vi "S4GUI_002.vi"(7 "Tab ObsEng":enum32{"Obs", "CCD modes", "Eng"}(tab)) -> ()   [LabVIEW 2018] (continued)
    tunnel: [_ _ _ w73] -> w5
    frame #0 {
      w37 = T12."Disabled and Grayed Out" ("Disabled")
      (unwired) u32 240 ("Tab Control Pane Dimension:Width")
      (unwired) u32 300 ("Tab Control Pane Dimension:Height")
      n2 = disable-structure shown="Enabled" {
        disable-tunnel: u32 211 ("Tab Control Pane Dimension:Height") -> [w46 _]
        disable-tunnel: u32 225 ("Tab Control Pane Dimension:Width") -> [w45 _]
        disable-tunnel: w36 -> [w44 _]
        disable-tunnel: w36 -> [w43 _]
        disable-tunnel: w36 -> [w42 _]
        disable-tunnel: w36 -> [w41 _]
        frame Enabled {
          n3 = property on="Tab CH1" class="TabCtl (strict)"(error in=w44, "PaneHeight"=w46, "PaneWidth"=w45) -> ()  [unwired: 1 in, 2 out]
          n4 = property on="Tab CH2" class="TabCtl (strict)"(error in=w43, "PaneHeight"=w46, "PaneWidth"=w45) -> ()  [unwired: 1 in, 2 out]
          n5 = property on="Tab CH3" class="TabCtl (strict)"(error in=w42, "PaneHeight"=w46, "PaneWidth"=w45) -> ()  [unwired: 1 in, 2 out]
          n6 = property on="Tab CH4" class="TabCtl (strict)"(error in=w41, "PaneHeight"=w46, "PaneWidth"=w45) -> ()  [unwired: 1 in, 2 out]
        }
        frame Disabled {
        }
      }
      n7 = local write "loop max(ms)"(u32 0 ("loop max(ms)")) -> ()
      n8 = property on="Set from Input ch1" class="Bool"(error in=w36, "DisabledEnum"=w37) -> ()  [unwired: 1 in, 2 out]
      n9 = property on="Set from Input ch3" class="Bool"(error in=w36, "DisabledEnum"=w37) -> ()  [unwired: 1 in, 2 out]
      n10 = property on="Set from Input ch2" class="Bool"(error in=w36, "DisabledEnum"=w37) -> ()  [unwired: 1 in, 2 out]
      n11 = property on="Set from Input ch4" class="Bool"(error in=w36, "DisabledEnum"=w37) -> (error out=w35:errorcluster)  [unwired: 1 in, 1 out]
    }
    frame #1 {
      w48 = u16 0 items=["OFF", "Lambda/2", "Lambda/4"] ("Lambda Selector")
      w52 = TRUE ("CH1on")
      w56 = u16 1 items=["Asynchronous", "Synchronous by Cycle"] ("SSM")
      w55 = u16 4 items=["All 16 positions", "First 8 positions", "First 4 positions", "1-4 & 9-12", "Clear", "Customized"] ("Select Positions")
      n12 = property on="#Pol. Seq. Done" class="Slide (strict)"(error in=w51, "Scale.Maximum"=0.0 ("Scale.Range:Maximum"), "Scale.Minimum"=0.0 ("Scale.Range:Minimum")) -> (error out=w50:errorcluster)  [unwired: 1 in, 1 out]
      n13 = local write "Tab ObsEng"(enum32{"Obs", "CCD modes", "Eng"}."Obs" ("Tab ObsEng")) -> ()
      n14 = property on="Tab ObsEng" class="TabCtl (strict)"(error in=w51, "Visible"=TRUE) -> ()  [unwired: 1 in, 2 out]
      n15 = property on="S4ICS protocol" class="Bool (strict)"(error in=w51, "Value"=FALSE ("S4ICS protocol"), "DisabledEnum"=T12."Disabled and Grayed Out" ("Disabled")) -> ()  [unwired: 1 in, 2 out]
      n16 = property on="SSM" class="Ring (strict)"(error in=w51, "Value"=w56) -> ()  [unwired: 1 in, 2 out]
      n17 = property on="TCS mode" class="Bool (strict)"(error in=w51, "Value"=TRUE ("TCS mode"), "DisabledEnum"=T12."Disabled and Grayed Out" ("Disabled")) -> ()  [unwired: 1 in, 2 out]
      n18 = property on="Lambda Selector" class="Ring (strict)"("Value"=w48) -> (error out=w49:errorcluster)  [unwired: 2 in, 1 out]
      n19 = local write "Select Positions"(w55) -> ()
      n20 = local write "password 2"("" ("password")) -> ()
      n21 = local write "password"("" ("password")) -> ()
      n22 = local write "CH2on"(w52) -> ()
      n23 = local write "CH3 on"(w52) -> ()
      n24 = local write "CH4 on"(w52) -> ()
      n25 = local write "CH1on"(w52) -> ()
      n26 = property on="Lambda Selector" class="Ring (strict)"(error in=w49, "RingText.Text"="Select...") -> ()  [unwired: 1 in, 2 out]
    }
    frame #2 {
      w69 = FALSE
      w66 = FALSE ("Cooler status 1")
      w65 = "" ("Temp Status 1")
      w70 = i16 0 ("Curr Temp 1")
      n27 = local write "Cooler status 4"(w66) -> ()
      n28 = local write "Curr Temp 4"(w70) -> ()
      n29 = local write "Panel Temp 4"(w70) -> ()
      n30 = local write "Temp Status 4"(w65) -> ()
      n31 = local write "Panel cooler 1"(w66) -> ()
      n32 = local write "Panel cooler 4"(w66) -> ()
      n33 = local write "Cooler status 1"(w66) -> ()
      n34 = local write "Curr Temp 1"(w70) -> ()
      n35 = local write "Panel Temp"(w70) -> ()
      n36 = local write "Temp Status 1"(w65) -> ()
      n37 = local write "Temp Status 3"(w65) -> ()
      n38 = local write "Panel Temp 3"(w70) -> ()
      n39 = local write "Panel cooler 2"(w66) -> ()
      n40 = local write "Curr Temp 2"(w70) -> ()
      n41 = local write "Panel Temp 2"(w70) -> ()
      n42 = local write "Temp Status 2"(w65) -> ()
      n43 = local write "Panel cooler 3"(w66) -> ()
      n44 = local write "Cooler status 3"(w66) -> ()
      n45 = local write "Cooler status 2"(w66) -> ()
      n46 = local write "Curr Temp 3"(w70) -> ()
      n47 = local write "P8"(w69) -> ()
      n48 = local write "P9"(w69) -> ()
      n49 = local write "P10"(w69) -> ()
      n50 = local write "P11"(w69) -> ()
      n51 = local write "P12"(w69) -> ()
      n52 = local write "P13"(w69) -> ()
      n53 = local write "P14"(w69) -> ()
      n54 = local write "P15"(w69) -> ()
      n55 = local write "P1"(w69) -> ()
      n56 = local write "P2"(w69) -> ()
      n57 = local write "P3"(w69) -> ()
      n58 = local write "P4"(w69) -> ()
      n59 = local write "P5"(w69) -> ()
      n60 = local write "P6"(w69) -> ()
      n61 = local write "P7"(w69) -> ()
      n62 = local write "P0"(TRUE ("P0")) -> ()
    }
    frame #3 {
      w91 = T12."Disabled" ("Disabled")
      n63 = property on="Observer" class="Str"(error in=w82, "Value"="" ("Observer"), "Text.BGColor"=u32 16448250) -> (error out=w78:errorcluster)  [unwired: 1 in, 1 out]
      n64 = property on="Project ID" class="Str"(error in=w82, "Value"="" ("Observer"), "Text.BGColor"=u32 16448250) -> ()  [unwired: 1 in, 2 out]
      n65 = property on="SendExpose" class="Bool (strict)"(error in=w82, "Value"=TRUE ("ExtSync")) -> ()  [unwired: 1 in, 2 out]
      n66 = property on="suffix alert" class="Str"(error in=w82, "Text.BGColor"=u32 16711680, "Text.TextColor"=u32 16776722) -> ()  [unwired: 1 in, 2 out]
      n67 = property on="Object_dflat" class="Str"(error in=w82, "DisabledEnum"=w91) -> ()  [unwired: 1 in, 2 out]
      n68 = property on="Object_zero" class="Str"(error in=w82, "DisabledEnum"=w91) -> ()  [unwired: 1 in, 2 out]
      n69 = property on="Object_sflat" class="Str"(error in=w82, "DisabledEnum"=w91) -> ()  [unwired: 1 in, 2 out]
      n70 = local write "GUIDER"(FALSE ("GUIDER")) -> ()
      n71 = property on="dark suffix" class="Str"(error in=w78, "Text.BGColor"=u32 16448250) -> ()  [unwired: 1 in, 2 out]
      n72 = property on="object suffix" class="Str"(error in=w78, "Text.BGColor"=u32 16448250) -> (error out=w74:errorcluster)  [unwired: 1 in, 1 out]
      n73 = property on="dflat suffix" class="Str"(error in=w78, "Text.BGColor"=u32 16448250) -> ()  [unwired: 1 in, 2 out]
      n74 = property on="SET Temp message" class="Bool (strict)"("Value"=TRUE ("SET Temp message")) -> ()  [unwired: 2 in, 2 out]
      n75 = property on="sflat suffix" class="Str"(error in=w74, "Text.BGColor"=u32 16448250) -> ()  [unwired: 1 in, 2 out]
      n76 = property on="zero suffix" class="Str"(error in=w74, "Text.BGColor"=u32 16448250) -> ()  [unwired: 1 in, 2 out]
      n77 = property on="focus suffix" class="Str"(error in=w74, "Text.BGColor"=u32 16448250) -> (error out=w73:errorcluster)  [unwired: 1 in, 1 out]
      "suffix alert" <- "Invalid char!" ("suffix alert")
      "FT warning" <- "" ("FT warning")
    }
  }
  n78 = disable-structure shown="Enabled" {
    disable-tunnel: "S4ACS_GUI.lvclass" -> [w100 w102]
    disable-tunnel: w5 -> [w99 w101]
    disable-tunnel: [w94 w102] -> w25
    disable-tunnel: [w93 w101] -> w24
    frame Enabled {
      # "Carrega o ultimo filtro escolhido para os 4 canais."
      n79 = local read "Filter1"() -> (w98:u8)
      n80 = local read "Filter2"() -> (w97:u8)
      n81 = local read "Filter3"() -> (w96:u8)
      n82 = local read "Filter4"() -> (w95:u8)
      n83 = call-dynamic "LoadFilters.vi"("Filter 4"=w95, "Filter 3"=w96, "error in (no error)"=w99, "Filter 2"=w97, "Filter 1"=w98, "S4GUI in"=w100) -> ("error out"=w93:errorcluster, "S4GUI out"=w94:refnum<class "S4GUI.lvclass">)  [unwired: 4 in]
    }
    frame Disabled {
    }
  }
  n84 = flat-sequence "Indicadores dos canais da parte inferior da tela principal" {
    frame #0 {
      w103 = ""
      "B1" <- w103
      "PA1" <- w103
      "RO1" <- w103
      "G1" <- w103
      "SI2" <- w103
      "PA2" <- w103
      "G2" <- w103
      "B2" <- w103
      "RO2" <- w103
      "EA2" <- w103
      "SI3" <- w103
      "EA3" <- w103
      "PA3" <- w103
      "B3" <- w103
      "G3" <- w103
      "RO3" <- w103
      "SI4" <- w103
      "EA4" <- w103
      "PA4" <- w103
      "B4" <- w103
      "G4" <- w103
      "RO4" <- w103
      "SI1" <- w103
      "EA1" <- w103
    }
  }
  n85 = call-dynamic "Write GUI version.vi"("error in (no error)"=w24, "GUI version"=w22, "S4GUI in"=w25) -> ("error out"=w16:errorcluster, "S4GUI out"=w23:refnum<class "S4GUI.lvclass">)  [unwired: 7 in]
  n86 = property on="Tab Acq Type" class="TabCtl (strict)"(error in=w16, "DisabledEnum"=T12."Disabled and Grayed Out" ("Disabled")) -> (error out=w15:errorcluster)  [unwired: 1 in, 1 out]
  n87 = control-ref of="Current Configuration"() -> (w33:refnum<vi>)
  n88 = control-ref of="Parameters"() -> (w30:refnum<vi>)
  n89 = call-dynamic "Initialize.vi"("error in (no error)"=w15, "S4ACS_GUI in"=w23) -> ("error out"=w14:errorcluster, "S4ACS_GUI out"=w18:refnum<class "S4GUI.lvclass">)  [unwired: 8 in]
  n90 = property on="Tab Acq Type" class="TabCtl (strict)"(error in=w14, "DisabledEnum"=T12."Enabled" ("Disabled")) -> (error out=w13:errorcluster)  [unwired: 1 in, 1 out]
  n91 = property on="Property Node" class="Clust (strict)"(reference=w30, "Top"=230 ("Position:Top")) -> (reference out=w34:refnum<vi>)  [unwired: 1 in, 1 out]
  n92 = property on="Property Node" class="Clust (strict)"(reference=w33, "Top"=230 ("Position:Top")) -> (reference out=w32:refnum<vi>)  [unwired: 1 in, 1 out]
  n93 = call-dynamic "Read TabAcqType index.vi"("error in (no error)"=w13, "S4GUI in"=w18) -> ("error out"=w10:errorcluster, "TabAcqType index"=w17:u32, "S4GUI out"=w11:refnum<class "S4GUI.lvclass">)  [unwired: 7 in]
  n94 = case shown="4" w17 {
    tunnel: [T1."OBJECT" ("Tab Acq Type") T1."DFLAT" ("Tab Acq Type") T1."SFLAT" ("Tab Acq Type") T1."DARK" ("Tab Acq Type") T1."ZERO" ("Tab Acq Type") T1."FOCUS" ("Tab Acq Type")] -> w7
    frame 0, Default {
    }
    frame 1 {
    }
    frame 2 {
    }
    frame 3 {
    }
    frame 4 {
      w108 = 1e-05 ("Exptime ch1")
      n95 = property on="Exptime ch1" class="DigNum (strict)"("Value"=w108) -> ()  [unwired: 2 in, 2 out]
      n96 = property on="Exptime ch2" class="DigNum (strict)"("Value"=w108) -> ()  [unwired: 2 in, 2 out]
      n97 = property on="Exptime ch3" class="DigNum (strict)"("Value"=w108) -> ()  [unwired: 2 in, 2 out]
      n98 = property on="Exptime ch4" class="DigNum (strict)"("Value"=w108) -> ()  [unwired: 2 in, 2 out]
    }
    frame 5 {
    }
  }
  n99 = local write "Tab Acq Type"(w7) -> ()
  n100 = Bundle("Parameters"=w34, "Current Configuration"=w32) -> (w31:T13)  [unwired: 1 in]
  n101 = call-dynamic "Write ExpMode.vi"("error in (no error)"=w10, "ExpMode"=w7, "S4GUI in"=w11) -> ("error out"=w9:errorcluster, "S4GUI out"=w8:refnum<class "S4GUI.lvclass">)  [unwired: 7 in]
  n102 = while {
    shift-right: [w129] -> w4
    shift-left: w8 -> [w131]
    shift-right: [w116] -> w2
    shift-left: w9 -> [w112]
    tunnel: w31 -> [w136]
    i -> [w122]
    stop <- w113 stop-if-true
    # "Sufixo do arquivo SEMPRE\nem minúsculas."
    n103 = case shown="\"OBJECT\", Default" "Tab Acq Type" {
      tunnel: ["object suffix" "dflat suffix" "sflat suffix" "dark suffix" "zero suffix" "focus suffix"] -> w124
      tunnel: ["OBJECT Comments" "DFLAT Comments" "SFLAT Comments" "DARK Comments" "ZERO Comments" "FOCUS Comments"] -> w137
      tunnel: ["OBJECT" "FLAT" "FLAT" "DARK" "ZERO" "FOCUS"] -> w134
      tunnel: ["Object_obj" "DOMEFLAT" "SKYFLAT" "Object_dark" "ZERO" "Object_focus"] -> w133
      tunnel: [_ _ _ _ _ "Start focus"] -> w121
      tunnel: [_ _ _ _ _ "Step focus"] -> w119
      tunnel: [_ _ _ _ _ "#steps"] -> w120
      frame "OBJECT", Default {
        (unwired) "" ("object suffix Temp")
      }
      frame "DFLAT" {
      }
      frame "SFLAT" {
      }
      frame "DARK" {
      }
      frame "ZERO" {
      }
      frame "FOCUS" {
      }
    }
    n104 = flat-sequence {
      tunnel: w131 -> [w151]
      tunnel: [w151] -> w111
      tunnel: [w150] -> w128
      frame #0 {
        n105 = case shown="False" "reset max" {
          frame False {
          }
          frame True {
            n106 = local write "loop max(ms)"(u32 0 ("loop max(ms)")) -> ()
          }
        }
        n107 = Tick Count (ms)() -> (millisecond timer value=w150:u32)
      }
    }
    n108 = To Lower Case(string=w124) -> (all lower case string=w123:string)
    n109 = event shown="[0] Timeout" {
      selector: _ -> [_ _ _ _ _ _ _ _ _ _ _ _ _ _ _ _ _ _ _ _ _ _ _ _ _ _ _ _ _ _ _ _ _ _ _ _ _ _ _ _ _ _ _ _ _ _ _ _ _ _ _ _ _ _ _ _ _ _ _ _ _ _ _ _ _ _ _ _ _ _ _ _ _ _ _ _ _ _ _ _ _ _ _ _ _ _ _ _ _ _ _ _ _ _ _ _ _ _ _ _ _ _ _ _ _ _ _ _ _ _ _ _ _ _ _ _ _ _ _ _ _ _ _ _ _ _ _ _ _ _ _ _ _ _ _ _]
      dyn-events: _ -> [_ _ _ _ _ _ _ _ _ _ _ _ _ _ _ _ _ _ _ _ _ _ _ _ _ _ _ _ _ _ _ _ _ _ _ _ _ _ _ _ _ _ _ _ _ _ _ _ _ _ _ _ _ _ _ _ _ _ _ _ _ _ _ _ _ _ _ _ _ _ _ _ _ _ _ _ _ _ _ _ _ _ _ _ _ _ _ _ _ _ _ _ _ _ _ _ _ _ _ _ _ _ _ _ _ _ _ _ _ _ _ _ _ _ _ _ _ _ _ _ _ _ _ _ _ _ _ _ _ _ _ _ _ _ _ _]
      timeout: 20 -> [_ _ _ _ _ _ _ _ _ _ _ _ _ _ _ _ _ _ _ _ _ _ _ _ _ _ _ _ _ _ _ _ _ _ _ _ _ _ _ _ _ _ _ _ _ _ _ _ _ _ _ _ _ _ _ _ _ _ _ _ _ _ _ _ _ _ _ _ _ _ _ _ _ _ _ _ _ _ _ _ _ _ _ _ _ _ _ _ _ _ _ _ _ _ _ _ _ _ _ _ _ _ _ _ _ _ _ _ _ _ _ _ _ _ _ _ _ _ _ _ _ _ _ _ _ _ _ _ _ _ _ _ _ _ _ _]
      tunnel: w111 -> [w189 w1985 w1996 w2001 w2006 w2011 w2016 w2021 w2291 w2450 w2480 w2486 w2508 w2530 w2716 w2724 w2803 w2824 w2896 w2967 w3068 w3082 w3223 w3462 w3494 w3526 w3558 w3593 w3628 w3663 w3698 w3701 w3735 w3877 w3938 w4445 w4524 w4596 w4667 w4740 w4791 w4832 w5261 w5267 w5387 w6719 w6862 w7067 w7255 w7519 w7738 w7753 w7961 w8123 w8290 w8457 w8616 w8636 w8656 w8676 w8697 w8762 w8827 w8892 w8957 w8994 w9022 w9050 w9079 w9152 w9282 w9316 w9375 w9434 w9493 w9552 w9572 w9599 w9615 w9636 w9666 w9696 w9721 w9762 w9803 w9844 w9885 w9926 w9967 w10008 w10051 w10166 w10276 w10386 w10495 w10505 w10525 w10540 w10555 w10570 w10585 w10600 w10615 w10630 w10661 w10690 w10714 w10756 w10790 w10817 w10840 w10868 w10888 w10903 w10923 w11006 w11334 w11360 w11514 w11534 w11549 w11569 w11589 w11609 w11624 w11644 w11664 w11684 w11699 w11719 w11739 w11759 w11774 w11794 w11814 w11834]
      tunnel: w112 -> [w188 w1984 w1995 w2000 w2005 w2010 w2015 w2020 w2292 w2448 w2479 w2485 w2507 w2529 w2715 w2723 w2802 w2823 w2895 w2968 w3067 w3074 w3219 w3461 w3493 w3525 w3557 w3592 w3627 w3662 w3697 w3709 w3736 w3876 w3937 w4444 w4523 w4595 w4663 w4739 w4789 w4831 w5260 w5266 w5386 w6718 w6861 w7066 w7254 w7512 w7736 w7752 w7959 w8122 w8288 w8456 w8617 w8637 w8657 w8677 w8696 w8761 w8826 w8891 w8955 w8992 w9020 w9048 w9078 w9151 w9281 w9315 w9374 w9433 w9492 w9551 w9571 w9598 w9614 w9635 w9665 w9695 w9720 w9761 w9802 w9843 w9884 w9925 w9966 w10007 w10050 w10165 w10275 w10385 w10494 w10504 w10524 w10539 w10554 w10569 w10584 w10599 w10614 w10629 w10660 w10689 w10713 w10755 w10789 w10816 w10839 w10867 w10887 w10902 w10922 w11007 w11333 w11359 w11513 w11533 w11548 w11568 w11588 w11608 w11623 w11643 w11663 w11683 w11698 w11718 w11738 w11758 w11773 w11793 w11813 w11833]
      tunnel: [w185 w1983 w1993 w1997 w2002 w2007 w2012 w2017 w2254 w2442 w2467 w2487 w2509 w2531 w2703 w2741 w2802 w2841 w2913 w2985 w3054 w3080 w3221 w3372 w3480 w3512 w3544 w3583 w3618 w3653 w3688 w3709 w3721 w3841 w3925 w4364 w4521 w4593 w4658 w4737 w4792 w4826 w5259 w5263 w5354 w6776 w6855 w7060 w7266 w7513 w7737 w7745 w7955 w8132 w8299 w8466 w8615 w8635 w8655 w8675 w8695 w8760 w8825 w8890 w8956 w8993 w9021 w9049 w9083 w9156 w9283 w9314 w9373 w9432 w9491 w9550 w9570 w9597 w9613 w9634 w9664 w9694 w9723 w9764 w9805 w9846 w9887 w9928 w9969 w10010 w10049 w10164 w10274 w10384 w10491 w10503 w10523 w10538 w10553 w10568 w10583 w10598 w10613 w10628 w10645 w10687 w10712 w10754 w10788 w10815 w10838 w10850 w10870 w10890 w10906 w10930 w11341 w11364 w11496 w11516 w11536 w11554 w11571 w11591 w11611 w11627 w11646 w11666 w11686 w11702 w11721 w11741 w11761 w11777 w11796 w11816] -> w116
      tunnel: [w186 _ _ _ _ _ _ _ _ _ _ _ _ _ _ _ _ _ _ _ _ _ _ _ _ _ _ _ _ _ _ _ _ _ _ _ _ _ _ _ _ _ _ _ _ _ _ _ _ _ _ _ _ _ _ _ _ _ _ _ _ _ _ _ _ _ _ _ _ _ _ _ _ _ _ _ _ _ _ _ _ _ _ _ _ _ _ _ _ _ _ _ _ _ _ _ _ _ _ _ _ _ _ _ _ _ _ _ _ _ _ _ _ _ _ _ _ _ _ _ _ _ _ _ _ _ _ _ _ _ _ _ _ _ _ _] -> w114
      tunnel: w123 -> [_ _ _ _ _ _ _ _ _ _ _ _ _ _ _ _ _ _ _ _ _ _ _ _ _ _ _ _ _ _ _ _ _ _ _ _ _ _ _ _ _ w4825 _ _ _ _ w6860 w7064 _ w7517 _ w7750 w7968 w8131 w8298 w8465 _ _ _ _ _ _ _ _ _ _ _ _ _ _ _ _ _ _ _ _ _ _ _ _ _ _ _ _ _ _ _ _ _ _ _ _ _ _ _ _ _ _ _ _ _ _ _ _ _ _ _ _ _ _ _ _ _ _ _ _ _ _ _ _ _ _ _ _ _ _ _ _ _ _ _ _ _ _ _ _]
      tunnel: w137 -> [_ _ _ _ _ _ _ _ _ _ _ _ _ _ _ _ _ _ _ _ _ _ _ _ _ _ _ _ _ _ _ _ _ _ _ _ _ _ _ _ _ w4824 _ _ _ _ w6859 _ w7270 w7516 _ w7749 w7967 w8130 w8297 w8464 _ _ _ _ _ _ _ _ _ _ _ _ _ _ _ _ _ _ _ _ _ _ _ _ _ _ _ _ _ _ _ _ _ _ _ _ _ _ _ _ _ _ _ _ _ _ _ _ _ _ _ _ _ _ _ _ _ _ _ _ _ _ _ _ _ _ _ _ _ _ _ _ _ _ _ _ _ _ _ _]
      tunnel: w136 -> [_ _ _ _ _ _ _ _ _ _ _ _ _ _ _ _ _ _ _ _ _ _ _ _ _ _ _ _ _ _ _ w3702 _ _ _ _ _ _ _ _ _ _ _ _ _ _ _ _ _ _ _ _ _ _ _ _ _ _ _ _ _ _ _ _ _ _ _ _ _ _ _ _ _ _ _ _ _ _ _ _ _ _ _ _ _ _ _ _ _ _ _ _ _ _ _ _ _ _ _ _ _ _ _ _ _ _ _ _ _ _ _ _ _ _ _ _ _ _ _ _ _ _ _ _ _ _ _ _ _ _ _ _ _ _ _ _]
      tunnel: [w184 w1985 w1994 w1998 w2003 w2008 w2013 w2018 w2256 w2441 w2468 w2488 w2510 w2532 w2704 w2742 w2803 w2842 w2914 w2986 w3045 w3081 w3222 w3374 w3471 w3503 w3535 w3560 w3595 w3630 w3665 w3701 w3720 w3842 w3926 w4365 w4522 w4594 w4659 w4738 w4793 w4806 w5258 w5262 w5355 w6775 w6856 w7061 w7267 w7514 w7738 w7746 w7956 w8129 w8296 w8463 w8614 w8634 w8654 w8674 w8694 w8759 w8824 w8889 w8954 w8991 w9019 w9047 w9081 w9154 w9284 w9313 w9372 w9431 w9490 w9549 w9569 w9589 w9612 w9633 w9663 w9693 w9722 w9763 w9804 w9845 w9886 w9927 w9968 w10009 w10048 w10163 w10273 w10383 w10492 w10496 w10519 w10534 w10549 w10564 w10579 w10594 w10609 w10624 w10644 w10662 w10699 w10723 w10771 w10801 w10826 w10849 w10869 w10889 w10904 w10931 w11342 w11365 w11495 w11515 w11535 w11552 w11570 w11590 w11610 w11625 w11645 w11665 w11685 w11700 w11720 w11740 w11760 w11775 w11795 w11815] -> w130
      tunnel: "Input Cluster" -> [_ _ _ _ _ _ _ _ _ _ _ _ _ _ _ _ _ _ _ _ _ _ _ _ _ _ _ _ _ _ _ w3700 _ _ _ _ _ _ _ _ _ _ _ _ _ _ _ _ _ _ _ _ _ _ _ _ _ _ _ _ _ _ _ _ _ _ _ _ _ _ _ _ _ _ _ _ _ _ _ _ _ _ _ _ _ _ _ _ _ _ _ _ _ _ _ _ _ _ _ _ _ _ _ _ _ _ _ _ _ _ _ _ _ _ _ _ _ _ _ _ _ _ _ _ _ _ _ _ _ _ _ _ _ _ _ _]
      tunnel: w134 -> [_ _ _ _ _ _ _ _ _ _ _ _ _ _ _ _ _ _ _ _ _ _ _ _ _ _ _ _ _ _ _ _ _ _ _ _ _ _ _ _ _ w4823 _ _ _ _ w6857 w7062 w7268 w7515 _ w7747 w7966 w8128 w8294 w8462 _ _ _ _ _ _ _ _ _ _ _ _ _ _ _ _ _ _ _ _ _ _ _ _ _ _ _ _ _ _ _ _ _ _ _ _ _ _ _ _ _ _ _ _ _ _ _ _ _ _ _ _ _ _ _ _ _ _ _ _ _ _ _ _ _ _ _ _ _ _ _ _ _ _ _ _ _ _ _ _]
      tunnel: w133 -> [_ _ _ _ _ _ _ _ _ _ _ _ _ _ _ _ _ _ _ _ _ _ _ _ _ _ _ _ _ _ _ _ _ _ _ _ _ _ _ _ _ w4822 _ _ _ _ _ w7065 w7271 w7518 _ w7751 w7965 w8127 w8295 w8461 _ _ _ _ _ _ _ _ _ _ _ _ _ _ _ _ _ _ _ _ _ _ _ _ _ _ _ _ _ _ _ _ _ _ _ _ _ _ _ _ _ _ _ _ _ _ _ _ _ _ _ _ _ _ _ _ _ _ _ _ _ _ _ _ _ _ _ _ _ _ _ _ _ _ _ _ _ _ _ _]
      tunnel: "Observer" -> [_ _ _ _ _ _ _ _ _ _ _ _ _ _ _ _ _ _ _ _ _ _ _ _ _ _ _ _ _ _ _ _ _ _ _ _ _ _ _ _ _ w4821 _ _ w5360 w6728 w6858 w7063 w7269 _ _ w7748 w7964 w8126 w8293 w8460 _ _ _ _ _ _ _ _ _ _ _ _ _ _ _ _ _ _ _ _ _ _ _ _ _ _ _ _ _ _ _ _ _ _ _ _ _ _ _ _ _ _ _ _ _ _ _ _ _ _ _ _ _ _ _ _ _ _ _ _ _ _ _ _ _ _ _ _ _ _ _ _ _ _ _ _ _ _ _ _]
      tunnel: w122 -> [w187 _ _ _ _ _ _ _ _ _ _ _ _ _ _ _ _ _ _ _ _ _ _ _ _ _ _ _ _ _ _ _ _ _ _ _ _ _ _ _ _ _ _ _ _ _ _ _ _ _ _ _ _ _ _ _ _ _ _ _ _ _ _ _ _ _ _ _ _ _ _ _ _ _ _ _ _ _ _ _ _ _ _ _ _ _ _ _ _ _ _ _ _ _ _ _ _ _ _ _ _ _ _ _ _ _ _ _ _ _ _ _ _ _ _ _ _ _ _ _ _ _ _ _ _ _ _ _ _ _ _ _ _ _ _ _]
      tunnel: "Tab Acq Type" -> [_ _ _ _ _ _ _ _ _ _ _ _ _ _ _ _ _ _ _ _ _ _ _ _ _ _ _ _ _ _ _ _ _ _ _ _ _ _ _ _ _ w4813 _ _ _ _ _ _ w7257 _ _ _ w7953 w8117 w8284 w8450 _ _ _ _ _ _ _ _ _ _ _ _ _ _ _ _ _ _ _ _ _ _ _ _ _ _ _ _ _ _ _ _ _ _ _ _ _ _ _ _ _ _ _ _ _ _ _ _ _ _ _ _ _ _ _ _ _ _ _ _ _ _ _ _ _ _ _ _ _ _ _ _ _ _ _ _ _ _ _ _]
      tunnel: w121 -> [_ _ _ _ _ _ _ _ _ _ _ _ _ _ _ _ _ _ _ _ _ _ _ _ _ _ _ _ _ _ _ _ _ _ _ _ _ _ _ _ _ w4812 _ _ _ _ _ _ _ _ _ _ w7952 w8116 w8283 w8449 _ _ _ _ _ _ _ _ _ _ _ _ _ _ _ _ _ _ _ _ _ _ _ _ _ _ _ _ _ _ _ _ _ _ _ _ _ _ _ _ _ _ _ _ _ _ _ _ _ _ _ _ _ _ _ _ _ _ _ _ _ _ _ _ _ _ _ _ _ _ _ _ _ _ _ _ _ _ _ _]
      tunnel: w120 -> [_ _ _ _ _ _ _ _ _ _ _ _ _ _ _ _ _ _ _ _ _ _ _ _ _ _ _ _ _ _ _ _ _ _ _ _ _ _ _ _ _ w4810 _ _ _ _ _ _ _ _ _ _ w7950 w8114 w8281 w8447 _ _ _ _ _ _ _ _ _ _ _ _ _ _ _ _ _ _ _ _ _ _ _ _ _ _ _ _ _ _ _ _ _ _ _ _ _ _ _ _ _ _ _ _ _ _ _ _ _ _ _ _ _ _ _ _ _ _ _ _ _ _ _ _ _ _ _ _ _ _ _ _ _ _ _ _ _ _ _ _]
      tunnel: w119 -> [_ _ _ _ _ _ _ _ _ _ _ _ _ _ _ _ _ _ _ _ _ _ _ _ _ _ _ _ _ _ _ _ _ _ _ _ _ _ _ _ _ w4811 _ _ _ _ _ _ _ _ _ _ w7951 w8115 w8282 w8448 _ _ _ _ _ _ _ _ _ _ _ _ _ _ _ _ _ _ _ _ _ _ _ _ _ _ _ _ _ _ _ _ _ _ _ _ _ _ _ _ _ _ _ _ _ _ _ _ _ _ _ _ _ _ _ _ _ _ _ _ _ _ _ _ _ _ _ _ _ _ _ _ _ _ _ _ _ _ _ _]
      tunnel: "Project ID" -> [_ _ _ _ _ _ _ _ _ _ _ _ _ _ _ _ _ _ _ _ _ _ _ _ _ _ _ _ _ _ _ _ _ _ _ _ _ _ _ _ _ _ _ _ w5359 w6727 _ _ _ _ _ _ _ _ _ _ _ _ _ _ _ _ _ _ _ _ _ _ _ _ _ _ _ _ _ _ _ _ _ _ _ _ _ _ _ _ _ _ _ _ _ _ _ _ _ _ _ _ _ _ _ _ _ _ _ _ _ _ _ _ _ _ _ _ _ _ _ _ _ _ _ _ _ _ _ _ _ _ _ _ _ _ _ _ _ _]
      event Timeout {
        # "execução do botão\nOK do SET TEMP de\ntodos os canais."
        # "2024.07.02: Mostra as publicações das aplicações."
        # "Trata as tarefas para atender \naos clientes: Publisher"
        # "Conteudo dos indicadores"
        # "Status dos indicadores: Habilitado ou Desab."
        # "Obtém os valores de status dos\ndispositivos de cada servidor para\napresentar nos indicadores da GUI."
        # "Trata as tarefas individuais de \ncada servidor (ACS1,...,ACS4, \nICS, TCS, Focus,Weather)"
        # "Determina a sequência de\ntarefas dos servidores\npara uma observação, de \nacordo com o modo de \noperação (disparado com \nos botões START)"
        # "execução dos botões\n no modo sincrono."
        # "execução dos botões\n no modo assincrono."
        n110 = event-data() -> ()  [unwired: 1 in, 2 out]
        n111 = disable-structure shown="Disabled" {
          disable-tunnel: w189 -> [w226 _]
          disable-tunnel: w188 -> [w224 _]
          frame Disabled {
            n112 = flat-sequence {
              tunnel: [w235] -> w225
              tunnel: w226 -> [w235]
              tunnel: w224 -> [w234]
              tunnel: [w234] -> w223
              frame #0 {
                n113 = local read "time alert"() -> (w232:u32)
                n114 = Tick Count (ms)() -> (millisecond timer value=w233:u32)
                n115 = Subtract(x=w233, y=w232) -> (x-y=w231:u32)
                n116 = Greater?(x=w231, y=u32 750) -> (0:w229:bool)
                n117 = case shown="True" w229 {
                  frame False {
                  }
                  frame True {
                    n118 = property on="suffix alert" class="Str"("Visible"=FALSE) -> ()  [unwired: 2 in, 2 out]
                  }
                }
              }
            }
            n119 = local read "charKeyboardInteger"() -> (w227:i16)
            n120 = call-dynamic "Read ExpMode.vi"("error in (no error)"=w223, "S4GUI in"=w225) -> ("ExpMode"=w228:T1)  [unwired: 7 in, 2 out]
            n121 = case shown="Default" w227 {
              tunnel: w228 -> [_ w237 w259]
              frame 32767 {
              }
              frame 0, 8, 32, 48..57, 65..90, 97..122 {
                n122 = case shown="\"OBJECT\", Default" w237 {
                  tunnel: [w242 w243 w244 w245 w246 w247] -> w238
                  frame "OBJECT", Default {
                    n123 = local read "object suffix"() -> (w242:string)
                  }
                  frame "DFLAT" {
                    n124 = local read "dflat suffix"() -> (w243:string)
                  }
                  frame "SFLAT" {
                    n125 = local read "sflat suffix"() -> (w244:string)
                  }
                  frame "DARK" {
                    n126 = local read "dark suffix"() -> (w245:string)
                  }
                  frame "ZERO" {
                    n127 = local read "zero suffix"() -> (w246:string)
                  }
                  frame "FOCUS" {
                    n128 = local read "focus suffix"() -> (w247:string)
                  }
                }
                n129 = String Length(string=w238) -> (length=w241:i32)
                n130 = Greater?(x=w241, y=10) -> (0:w239:bool)
                n131 = case shown="True" w239 {
                  tunnel: w238 -> [w248 _]
                  tunnel: w237 -> [_ w250]
                  frame False {
                    n132 = local write "suffix temp"(w248) -> ()
                  }
                  frame True {
                    n133 = local read "suffix temp"() -> (w249:string)
                    n134 = case shown="\"OBJECT\", Default" w250 {
                      tunnel: w249 -> [w251 w252 w253 w254 w255 w256]
                      frame "OBJECT", Default {
                        n135 = local write "object suffix"(w251) -> ()
                      }
                      frame "DFLAT" {
                        n136 = local write "dflat suffix"(w252) -> ()
                      }
                      frame "SFLAT" {
                        n137 = local write "sflat suffix"(w253) -> ()
                      }
                      frame "DARK" {
                        n138 = local write "dark suffix"(w254) -> ()
                      }
                      frame "ZERO" {
                        n139 = local write "zero suffix"(w255) -> ()
                      }
                      frame "FOCUS" {
                        n140 = local write "focus suffix"(w256) -> ()
                      }
                    }
                  }
                }
              }
              frame Default {
                n141 = local write "charKeyboardInteger"(i16 32767 ("lastChar")) -> ()
                n142 = Tick Count (ms)() -> (millisecond timer value=→"time alert":u32)
                n143 = property on="suffix alert" class="Str"("Visible"=TRUE) -> ()  [unwired: 2 in, 2 out]
                n144 = case shown="\"OBJECT\", Default" w259 {
                  tunnel: "suffix temp" -> [w262 w263 w264 w265 w266 w267]
                  frame "OBJECT", Default {
                    n145 = local write "object suffix"(w262) -> ()
                  }
                  frame "DFLAT" {
                    n146 = local write "dflat suffix"(w263) -> ()
                  }
                  frame "SFLAT" {
                    n147 = local write "sflat suffix"(w264) -> ()
                  }
                  frame "DARK" {
                    n148 = local write "dark suffix"(w265) -> ()
                  }
                  frame "ZERO" {
                    n149 = local write "zero suffix"(w266) -> ()
                  }
                  frame "FOCUS" {
                    n150 = local write "focus suffix"(w267) -> ()
                  }
                }
              }
            }
          }
          frame Enabled {
          }
        }
        n151 = disable-structure shown="Enabled" {
          disable-tunnel: w189 -> [w273 w278]
          disable-tunnel: w188 -> [w272 w276]
          disable-tunnel: [w270 w275] -> w181
          disable-tunnel: [w269 w274] -> w183
          disable-tunnel: w187 -> [_ w277]
          frame Disabled {
            n152 = call "Elapsed Time"() -> ("Time has Elapsed"=w268:bool)  [unwired: 12 in, 7 out]
            n153 = call "Elapsed Time3"() -> ("Time has Elapsed"=w271:bool)  [unwired: 12 in, 7 out]
            n154 = call "Write Status_timeout.vi"("error in (no error)"=w272, "TCS_timeout"=w271, "Status_timeout"=w268, "S4ACS_GUI in"=w273) -> ("error out"=w270:errorcluster, "S4ACS_GUI out"=w269:refnum<class "S4GUI.lvclass">)  [unwired: 6 in]
          }
          frame Enabled {
            n155 = call-dynamic "Write loop counter.vi"("error in (no error)"=w276, "loop counter"=w277, "S4GUI in"=w278) -> ("error out"=w275:errorcluster, "S4GUI out"=w274:refnum<class "S4GUI.lvclass">)  [unwired: 7 in]
          }
        }
        n156 = call-dynamic "HandleSetTemp.vi"("error in (no error)"=w181, "S4GUI in"=w183) -> ("error out"=w180:errorcluster, "S4GUI out"=w182:refnum<class "S4GUI.lvclass">)  [unwired: 8 in]
        n157 = call-dynamic "GetPubs.vi"("error in (no error)"=w180, "S4GUI in"=w182) -> ("error out"=w200:errorcluster, "Pubs out"=→"All Pubs":T11, "S4GUI out"=w199:refnum<class "S4GUI.lvclass">)  [unwired: 7 in]
        n158 = call-dynamic "HandlePauseAsync.vi"("error in (no error)"=w200, "S4GUI in"=w199) -> ("error out"=w217:errorcluster, "S4GUI out"=w219:refnum<class "S4GUI.lvclass">)  [unwired: 8 in]
        n159 = call-dynamic "HandleStopAsync.vi"("error in (no error)"=w217, "S4GUI in"=w219) -> ("error out"=w216:errorcluster, "S4GUI out"=w218:refnum<class "S4GUI.lvclass">)  [unwired: 8 in]
        n160 = call-dynamic "HandleAbortAsync.vi"("error in (no error)"=w216, "S4GUI in"=w218) -> ("error out"=w210:errorcluster, "S4GUI out"=w211:refnum<class "S4GUI.lvclass">)  [unwired: 8 in]
        n161 = call-dynamic "HandlePauseSync.vi"("error in (no error)"=w210, "S4GUI in"=w211) -> ("error out"=w209:errorcluster, "S4GUI out"=w208:refnum<class "S4GUI.lvclass">)  [unwired: 8 in]
        n162 = call-dynamic "HandleStopSync.vi"("error in (no error)"=w209, "S4GUI in"=w208) -> ("error out"=w213:errorcluster, "S4GUI out"=w215:refnum<class "S4GUI.lvclass">)  [unwired: 8 in]
        n163 = call-dynamic "HandleAbortSync.vi"("error in (no error)"=w213, "S4GUI in"=w215) -> ("error out"=w212:errorcluster, "S4GUI out"=w214:refnum<class "S4GUI.lvclass">)  [unwired: 8 in]
        n164 = call-dynamic "HandleObservation.vi"("error in (no error)"=w212, "S4ACS_GUI in"=w214) -> ("error out"=w221:errorcluster, "S4ACS_GUI out"=w222:refnum<class "S4GUI.lvclass">)  [unwired: 8 in]
        n165 = call-dynamic "HandleServers.vi"("error in (no error)"=w221, "S4GUI in"=w222) -> ("error out"=w203:errorcluster, "S4GUI out"=w204:refnum<class "S4GUI.lvclass">)  [unwired: 8 in]
        n166 = call-dynamic "HandleClients.vi"("error in (no error)"=w203, "S4GUI in"=w204) -> ("error out"=w202:errorcluster, "S4GUI out"=w194:refnum<class "S4GUI.lvclass">)  [unwired: 8 in]
        n167 = call-dynamic "GetStatus.vi"("error in (no error)"=w202, "S4GUI in"=w194) -> ("error out"=w196:errorcluster, "S4GUI out"=w193:refnum<class "S4GUI.lvclass">)  [unwired: 8 in]
        n168 = call-dynamic "Read output cluster.vi"("error in (no error)"=w196, "S4GUI in"=w193) -> ("error out"=w195:errorcluster, "output cluster"=w190:T15, "S4GUI out"=w192:refnum<class "S4GUI.lvclass">)  [unwired: 7 in]
        n169 = call "Elapsed Time2"() -> ("Time has Elapsed"=w207:bool)  [unwired: 12 in, 7 out]
        n170 = call-dynamic "Read Cluster Disable.vi"("error in (no error)"=w195, "S4GUI in"=w192) -> ("error out"=w197:errorcluster, "Cluster Disable"=w198:T16, "S4GUI out"=w191:refnum<class "S4GUI.lvclass">)  [unwired: 7 in]
        n171 = call "Read cfg file.vi"("error in (no error)"=w197, "S4ACS_GUI in"=w191) -> ("error out"=w205:errorcluster, "cfg file"=w220:string, "S4ACS_GUI out"=w206:refnum<class "S4GUI.lvclass">)  [unwired: 7 in]
        n172 = case shown="True" w207 {
          tunnel: w190 -> [_ w336]
          tunnel: w198 -> [_ w335]
          tunnel: w220 -> [_ w334]
          tunnel: w206 -> [w281 w333]
          tunnel: w205 -> [w280 w332]
          tunnel: [w280 w284] -> w185
          tunnel: [FALSE ("exit") w283] -> w186
          tunnel: [w281 w282] -> w184
          frame False {
          }
          frame True {
            w291 = "arking" ("regular expression")
            w309 = "ERRO" ("regular expression")
            # "Verifica mudança de modo e se deve carregar valores default \npara procedimento de ajuste de foco do telescópio."
            # "1a vez FOTOM (F)"
            # "1a vez POLAR (F)"
            # "MODE:\nF -> photometric\nT -> polarimetric"
            n173 = stacked-sequence {
              tunnel: w333 -> [w385 w392 w403 w413 w422]
              tunnel: w332 -> [w384 w391 w402 w412 w421]
              tunnel: [_ _ _ _ w420] -> w326
              tunnel: [_ _ _ _ w419] -> w325
              tunnel: [_ _ _ _ w418] -> w294
              frame #0 {
                n174 = call-dynamic "Read AcquisitionA.vi"("error in (no error)"=w384, "S4ACS_GUI in"=w385) -> ("error out"=w381:errorcluster, "Acquisition.lvclass"=w383:refnum<class "Acquisition.lvclass">)  [unwired: 7 in, 1 out]
                n175 = call-dynamic "Read Channel.vi"("error in (no error)"=w381, "Acquisition in"=w383) -> ("error out"=w380:errorcluster, "Channel.lvclass"=w382:refnum<class "Channel.lvclass">)  [unwired: 7 in, 1 out]
                n176 = call-dynamic "Read CyclesDone.vi"("error in (no error)"=w380, "Channel in"=w382) -> ("error out"=→"error out 6":errorcluster, "CyclesDone"=w377:u32)  [unwired: 7 in, 1 out]
                "Cycles Done ch1" <- w377
                n177 = Number To Decimal String(number=w377) -> (decimal integer string=w376:string)  [unwired: 1 in]
                n178 = Concatenate Strings("#Cycles Done ", w376) -> (w375:string)
                n179 = property on="Cycles Done ch1" class="Slide (strict)"("Caption.Text"=w375) -> ()  [unwired: 2 in, 2 out]
              }
              frame #1 {
                n180 = call "Read AcquisitionB.vi"("error in (no error)"=w391, "S4ACS_GUI in"=w392) -> ("error out"=w394:errorcluster, "Acquisition.lvclass"=w395:refnum<class "Acquisition.lvclass">)  [unwired: 7 in, 1 out]
                n181 = call-dynamic "Read Channel.vi"("error in (no error)"=w394, "Acquisition in"=w395) -> ("error out"=w393:errorcluster, "Channel.lvclass"=w396:refnum<class "Channel.lvclass">)  [unwired: 7 in, 1 out]
                n182 = call-dynamic "Read CyclesDone.vi"("error in (no error)"=w393, "Channel in"=w396) -> ("error out"=→"error out 4":errorcluster, "CyclesDone"=w387:u32)  [unwired: 7 in, 1 out]
                "Cycles Done ch2" <- w387
                n183 = Number To Decimal String(number=w387) -> (decimal integer string=w388:string)  [unwired: 1 in]
                n184 = Concatenate Strings("#Cycles Done ", w388) -> (w386:string)
                n185 = property on="Cycles Done ch2" class="Slide (strict)"("Caption.Text"=w386) -> ()  [unwired: 2 in, 2 out]
              }
              frame #2 {
                n186 = call-dynamic "Read AcquisitionC.vi"("error in (no error)"=w402, "S4ACS_GUI in"=w403) -> ("error out"=w405:errorcluster, "Acquisition.lvclass"=w406:refnum<class "Acquisition.lvclass">)  [unwired: 7 in, 1 out]
                n187 = call-dynamic "Read Channel.vi"("error in (no error)"=w405, "Acquisition in"=w406) -> ("error out"=w404:errorcluster, "Channel.lvclass"=w407:refnum<class "Channel.lvclass">)  [unwired: 7 in, 1 out]
                n188 = call-dynamic "Read CyclesDone.vi"("error in (no error)"=w404, "Channel in"=w407) -> ("error out"=→"error out 5":errorcluster, "CyclesDone"=w398:u32)  [unwired: 7 in, 1 out]
                "Cycles Done ch3" <- w398
                n189 = Number To Decimal String(number=w398) -> (decimal integer string=w399:string)  [unwired: 1 in]
                n190 = Concatenate Strings("#Cycles Done ", w399) -> (w397:string)
                n191 = property on="Cycles Done ch3" class="Slide (strict)"("Caption.Text"=w397) -> ()  [unwired: 2 in, 2 out]
              }
              frame #3 {
                n192 = call-dynamic "Read AcquisitionD.vi"("error in (no error)"=w412, "S4ACS_GUI in"=w413) -> ("error out"=w415:errorcluster, "Acquisition.lvclass"=w416:refnum<class "Acquisition.lvclass">)  [unwired: 7 in, 1 out]
                n193 = call-dynamic "Read Channel.vi"("error in (no error)"=w415, "Acquisition in"=w416) -> ("error out"=w414:errorcluster, "Channel.lvclass"=w417:refnum<class "Channel.lvclass">)  [unwired: 7 in, 1 out]
                n194 = call-dynamic "Read CyclesDone.vi"("error in (no error)"=w414, "Channel in"=w417) -> ("CyclesDone"=w409:u32)  [unwired: 7 in, 2 out]
                "Cycles Done ch4" <- w409
                n195 = Number To Decimal String(number=w409) -> (decimal integer string=w410:string)  [unwired: 1 in]
                n196 = Concatenate Strings("#Cycles Done ", w410) -> (w408:string)
                n197 = property on="Cycles Done ch4" class="Slide (strict)"("Caption.Text"=w408) -> ()  [unwired: 2 in, 2 out]
              }
              frame #4 {
                n198 = call-dynamic "Read SET request.vi"("error in (no error)"=w421, "S4GUI in"=w422) -> ("error out"=w419:errorcluster, "SET request"=w418:bool, "S4GUI out"=w420:refnum<class "S4GUI.lvclass">)  [unwired: 7 in]
              }
            }
            n199 = stacked-sequence {
              tunnel: w336 -> [w468 w478 w490 w492 w500 w546 w549 w683 w786 w1128 _ _ _ _ _ w1320 w1506 w1669 w1828 w1938]
              tunnel: [_ _ _ _ _ _ _ w681 _ _ _ _ _ _ _ _ _ _ _ _] -> w316
              tunnel: w335 -> [_ w474 _ _ _ _ _ _ _ _ w1155 w1202 w1219 w1236 w1253 _ _ _ _ _]
              tunnel: w334 -> [_ _ _ _ _ _ _ _ _ _ _ _ _ _ _ w1315 _ _ _ _]
              tunnel: w294 -> [_ _ _ _ _ _ _ _ _ _ _ _ _ _ _ _ _ _ _ w1941]
              frame #0 {
                (unwired) u32 240 ("Tab Control Pane Dimension:Width")
                (unwired) u32 300 ("Tab Control Pane Dimension:Height")
                n200 = Unbundle By Name(w468) -> ("GS STATUS cluster.AG"=→"GUIDER":bool, "TCS id"=w434:u32, "TCSPD_connection"=→"TCSPD":bool, "TCS extended"=w465:string, "focus pos"=w430:i32, "weather status"=w428:T17)
                n201 = Unbundle By Name(w428) -> ("outTemp"=→"Outside Temp":string, "pressure"=→"Pressure":string, "outHumidity"=→"Humidity":string, "windSpeed"=→"Wind Speed[Km/h]":string)
                n202 = Number To Decimal String(number=w430) -> (decimal integer string=→"Telescope Focus":string)  [unwired: 1 in]
                n203 = Equal?(x=u32 6 ("Tab Control Pane Dimension:Width"), y=w434) -> (x = y?=w433:bool)
                n204 = Match Pattern(string=w465, regular expression="RA=") -> (after substring=w461:string)  [unwired: 1 in, 3 out]
                n205 = local write "TCS mode"(w433) -> ()
                n206 = Match Pattern(string=w461, regular expression="DEC=") -> (before substring=→"RA":string, after substring=w460:string)  [unwired: 1 in, 2 out]
                n207 = Match Pattern(string=w460, regular expression="EQUINOX=") -> (before substring=→"DEC":string, after substring=w459:string)  [unwired: 1 in, 2 out]
                n208 = Match Pattern(string=w459, regular expression="AIRMASS=") -> (after substring=w455:string)  [unwired: 1 in, 3 out]
                n209 = Match Pattern(string=w455, regular expression="TCSHA=") -> (before substring=→"Air Mass":string, after substring=w454:string)  [unwired: 1 in, 2 out]
                n210 = Match Pattern(string=w454, regular expression="TCSDATE=") -> (before substring=→"Hour Angle":string, after substring=w452:string)  [unwired: 1 in, 2 out]
                n211 = Match Pattern(string=w452, regular expression="TELFOCUS=") -> (before substring=→"Date":string, after substring=w448:string)  [unwired: 1 in, 2 out]
                n212 = Match Pattern(string=w448, regular expression="EXTTEMP=") -> (after substring=w447:string)  [unwired: 1 in, 3 out]
                n213 = Match Pattern(string=w447, regular expression="PRESSURE=") -> (after substring=w446:string)  [unwired: 1 in, 3 out]
                n214 = Match Pattern(string=w446, regular expression="HUMIDITY=") -> (after substring=w438:string)  [unwired: 1 in, 3 out]
                n215 = Match Pattern(string=w438, regular expression="JD=") -> (after substring=w439:string)  [unwired: 1 in, 3 out]
                n216 = disable-structure shown="Enabled" {
                  disable-tunnel: u32 211 ("Tab Control Pane Dimension:Height") -> [w470 _]
                  disable-tunnel: u32 225 ("Tab Control Pane Dimension:Width") -> [w469 _]
                  frame Disabled {
                    n217 = property on="Tab CH1" class="TabCtl (strict)"("PaneHeight"=w470, "PaneWidth"=w469) -> ()  [unwired: 2 in, 2 out]
                    n218 = property on="Tab CH2" class="TabCtl (strict)"("PaneHeight"=w470, "PaneWidth"=w469) -> ()  [unwired: 2 in, 2 out]
                    n219 = property on="Tab CH3" class="TabCtl (strict)"("PaneHeight"=w470, "PaneWidth"=w469) -> ()  [unwired: 2 in, 2 out]
                    n220 = property on="Tab CH4" class="TabCtl (strict)"("PaneHeight"=w470, "PaneWidth"=w469) -> ()  [unwired: 2 in, 2 out]
                  }
                  frame Enabled {
                  }
                }
                n221 = Match Pattern(string=w439, regular expression="SD=") -> (before substring=→"Julian Date":string, after substring=→"Sideral Time":string)  [unwired: 1 in, 2 out]
              }
              frame #1 {
                # "OV 2024 09 04: Depois da criação da aba CCD modes, TODOS os parametros da aba Camera são protegidos por senha, \ninclusive as chaves de habilitação dos canais."
                n222 = Unbundle By Name(w478) -> ("S4ICS id"=w476:u32)
                n223 = Unbundle By Name(w474) -> ("Cluster AdmCCDsetup.param"=w471:T12)
                n224 = Equal?(x=u32 11, y=w476) -> (x = y?=w475:bool)
                n225 = local write "S4ICS protocol"(w475) -> ()
                n226 = case shown="\"Disabled and Grayed Out\"" w471 {
                  tunnel: [_ w480 w484] -> w473
                  frame Default {
                  }
                  frame "Disabled" {
                    n227 = Build Array(u32 4 ("element"), u32 5 ("element"), u32 6 ("element")) -> (w480:u32[])
                  }
                  frame "Disabled and Grayed Out" {
                    n228 = Build Array(u32 4 ("element"), u32 5 ("element"), u32 6 ("element")) -> (w484:u32[])
                  }
                }
                n229 = property on="Trigger\nMode" class="Ring (strict)"("DisabledEnum"=w471) -> ()  [unwired: 2 in, 2 out]
                n230 = property on="Vertical\nShift Speed" class="Ring (strict)"("DisabledEnum"=w471) -> ()  [unwired: 2 in, 2 out]
                n231 = property on="Vertical\nClock Voltage" class="Ring (strict)"("DisabledEnum"=w471) -> ()  [unwired: 2 in, 2 out]
                n232 = To Long Integer(number=w473) -> (32bit integer=w472:i32[])
                n233 = property on="EM Gain" class="DigNum (strict)"("DisabledEnum"=w471) -> ()  [unwired: 2 in, 2 out]
                n234 = property on="Read\nMode" class="Ring (strict)"("DisabledEnum"=w471) -> ()  [unwired: 2 in, 2 out]
                n235 = property on="AQM" class="Enum (strict)"("Disabled Items []"=w472) -> ()  [unwired: 2 in, 2 out]
                n236 = property on="Acquisition\nMode" class="Ring (strict)"("DisabledEnum"=w471) -> ()  [unwired: 2 in, 2 out]
                n237 = property on="A/D \nChannel" class="DigNum (strict)"("DisabledEnum"=w471) -> ()  [unwired: 2 in, 2 out]
                n238 = property on="Readout\nRate" class="Ring (strict)"("DisabledEnum"=w471) -> ()  [unwired: 2 in, 2 out]
                n239 = property on="CCD \nEM Mode" class="Ring (strict)"("DisabledEnum"=w471) -> ()  [unwired: 2 in, 2 out]
                n240 = property on="CCD\nEM Gain" class="DigNum (strict)"("DisabledEnum"=w471) -> ()  [unwired: 2 in, 2 out]
                n241 = property on="Shutter\nTTL" class="Ring (strict)"("DisabledEnum"=w471) -> ()  [unwired: 2 in, 2 out]
                n242 = property on="Shutter\nOpenning Time" class="DigNum (strict)"("DisabledEnum"=w471) -> ()  [unwired: 2 in, 2 out]
                n243 = property on="Frame\nTransfer" class="Bool (strict)"("DisabledEnum"=w471) -> ()  [unwired: 2 in, 2 out]
                n244 = property on="Shutter\nMode" class="Ring (strict)"("DisabledEnum"=w471) -> ()  [unwired: 2 in, 2 out]
                n245 = property on="Pre-amplification\nGain" class="Ring (strict)"("DisabledEnum"=w471) -> ()  [unwired: 2 in, 2 out]
                n246 = property on="Shutter\nClosing Time" class="DigNum (strict)"("DisabledEnum"=w471) -> ()  [unwired: 2 in, 2 out]
                n247 = property on="Horizontal\nBinning" class="DigNum (strict)"("DisabledEnum"=w471) -> ()  [unwired: 2 in, 2 out]
                n248 = property on="Vertical\nBinning" class="DigNum (strict)"("DisabledEnum"=w471) -> ()  [unwired: 2 in, 2 out]
                n249 = property on="Image\nFInal Column" class="DigNum (strict)"("DisabledEnum"=w471) -> ()  [unwired: 2 in, 2 out]
                n250 = property on="CH1on" class="Bool (strict)"("DisabledEnum"=w471) -> ()  [unwired: 2 in, 2 out]
                n251 = property on="CH2on" class="Bool (strict)"("DisabledEnum"=w471) -> ()  [unwired: 2 in, 2 out]
                n252 = property on="CH3 on" class="Bool (strict)"("DisabledEnum"=w471) -> ()  [unwired: 2 in, 2 out]
                n253 = property on="CH4 on" class="Bool (strict)"("DisabledEnum"=w471) -> ()  [unwired: 2 in, 2 out]
                n254 = property on="Image\nFinal Line" class="DigNum (strict)"("DisabledEnum"=w471) -> ()  [unwired: 2 in, 2 out]
                n255 = property on="Image\nInitial Column" class="DigNum (strict)"("DisabledEnum"=w471) -> ()  [unwired: 2 in, 2 out]
                n256 = property on="Image \nInitial Line" class="DigNum (strict)"("DisabledEnum"=w471) -> ()  [unwired: 2 in, 2 out]
              }
              frame #2 {
                n257 = Unbundle By Name(w490) -> ("Trigger Mode Status"=→"String":string, "Focus_connection"=→"Focus 160":bool, "WS_connection"=→"Weather":bool)
              }
              frame #3 {
                n258 = Unbundle By Name(w492) -> ("Trigger General Status"=→"String 2":string)
              }
              frame #4 {
                n259 = Unbundle By Name(w500) -> ("Instrument Motor error"=w493:T18, "Instrument Status"=w494:T19, "Instrument States.WPROT State"=w499:i32, "Instrument Pos Names.WPROT posname"=w498:string, "Instrument Pos Names.WPSEL posname"=w497:string, "Instrument Pos Names.CALW posname"=w496:string, "Instrument Pos Names.ASEL posname"=w495:string)
                n260 = stacked-sequence {
                  tunnel: w494 -> [w507 w512 w517 w521 w525 w530 w535 w541 w543]
                  tunnel: w499 -> [w503 _ _ _ _ _ _ _ _]
                  tunnel: w498 -> [_ w510 _ _ _ _ _ _ _]
                  tunnel: w497 -> [_ _ w515 _ _ _ _ _ _]
                  tunnel: w496 -> [_ _ _ _ _ w528 _ _ _]
                  tunnel: w495 -> [_ _ _ _ _ _ w533 _ _]
                  tunnel: w493 -> [_ w509 w514 w519 w523 w527 w532 _ _]
                  frame #0 {
                    # "Pisca quando BUSY"
                    n261 = Unbundle By Name(w507) -> ("WPROT pos"=w504:dbl)
                    "WaveplatePos 2" <- w504
                    n262 = Equal?(x=w503, y=3) -> (x = y?=w501:bool)
                    n263 = property on="WaveplatePos 2" class="DigNum (strict)"("Blinking"=w501) -> ()  [unwired: 2 in, 2 out]
                    n264 = Number To Fractional String(number=w504, precision (6)=i16 1) -> (F-format string=→"Angle":string)  [unwired: 2 in]
                  }
                  frame #1 {
                    n265 = Unbundle By Name(w509) -> ("WPROT error"=→"WPROT motor error":bool)
                    n266 = Unbundle By Name(w512) -> ("WPROT pos"=→"Position WPROT":dbl)
                    "PosName WPROT" <- w510
                  }
                  frame #2 {
                    n267 = Unbundle By Name(w517) -> ("WPSEL pos"=→"Position WPSEL":dbl)
                    n268 = Unbundle By Name(w514) -> ("WPSEL error"=→"WPSEL motor error":bool)
                    "PosName WPSEL" <- w515
                  }
                  frame #3 {
                    n269 = Unbundle By Name(w521) -> ("GMIR pos"=→"Position GMIR":dbl)
                    n270 = Unbundle By Name(w519) -> ("GMIR error"=→"GMIR motor error":bool)
                  }
                  frame #4 {
                    n271 = Unbundle By Name(w525) -> ("GFOC pos"=→"Position GFOC":dbl)
                    n272 = Unbundle By Name(w523) -> ("GFOC error"=→"GFOC motor error":bool)
                  }
                  frame #5 {
                    n273 = Unbundle By Name(w530) -> ("CALW pos"=→"Position CALW":dbl)
                    n274 = Unbundle By Name(w527) -> ("CALW error"=→"CALW motor error":bool)
                    "PosName CALW" <- w528
                  }
                  frame #6 {
                    n275 = Unbundle By Name(w535) -> ("ASEL pos"=→"PosName ASEL":dbl)
                    n276 = Unbundle By Name(w532) -> ("ASEL error"=→"ASEL motor error":bool)
                    "PosName ASEL" <- w533
                  }
                  frame #7 {
                    w537 = cluster{u32, u32}[] [{16711680, 16711680}, {15400704, 15400704}, {16776722, 0}, {16776722, 0}]  # amarelo
                    w536 = cluster{u32, u32}[] [{16711680, 16711680}, {6618880, 6618880}, {16776722, 0}, {16776722, 0}]  # verde
                    n277 = Unbundle By Name(w541) -> ("connection"=→"S4ICSoft":bool, "operational"=w539:bool)
                    n278 = Select(t=w536, s=w539, f=w537) -> (s? t:f=w538:cluster{u32, u32}[])
                    n279 = property on="S4ICSoft" class="Bool (strict)"("Colors [4]"=w538) -> ()  [unwired: 2 in, 2 out]
                  }
                  frame #8 {
                    n280 = Unbundle By Name(w543) -> ("String Status"=→"Status":string)
                  }
                }
              }
              frame #5 {
                n281 = Unbundle By Name(w546) -> ("Sync Box State"=→"Current State":i32, "Trigger_connection"=→"Sync Box" →"LedExtSync":bool)
              }
              frame #6 {
                # "Instrument States.<device> State\n\n0: nao fez INIT e está parado (mode = IDLE ou WAITING\n                                                    contdition = default)\n1: nao fez INIT e está movendo (mode = IDLE ou WAITING\n                                                    contdition = BUSY)\n\n2: fez INIT e está parado (mode = default)\n                                            condition = READY)\n3: fez INIT e está movendo (mode = default)\n                                            condition = BUSY)"
                n282 = Unbundle By Name(w549) -> ("Instrument States"=w548:T20, "Instrument Pos Names"=w547:T21)
                n283 = stacked-sequence {
                  tunnel: w548 -> [w557 w579 w597 w631 w660]
                  tunnel: w547 -> [w553 _ w595 w627 _]
                  frame #0 {
                    # "WPSEL"
                    n284 = Unbundle By Name(w553) -> ("WPSEL posname"=w550:string)
                    n285 = Unbundle By Name(w557) -> ("WPSEL State"=w556:i32)
                    n286 = local read "WPSEL Status"() -> (w552:bool)
                    n287 = case shown="2" w556 {
                      tunnel: [cluster{u32, u32}[] [{9868950, 9868950}, {9868950, 9868950}] ("Colors [4]") cluster{u32, u32}[] [{9868950, 9868950}, {9868950, 9868950}] ("Colors [4]") cluster{u32, u32}[] [{16318208, 16318208}, {16318208, 16318208}] ("Colors [4]") cluster{u32, u32}[] [{6618880, 2424594}, {6618880, 2424594}] ("Colors [4]") w571] -> w555
                      tunnel: [FALSE ("WPROT Status") FALSE ("WPROT Status") TRUE ("WPROT Status") FALSE ("WPROT Status") w573] -> w554
                      tunnel: w552 -> [_ _ _ _ w572]
                      tunnel: ["" "" "" w567 ""] -> w551
                      tunnel: w550 -> [_ _ _ w567 _]
                      frame Default {
                      }
